vi "MT Generate PSK System Parameters(M).vi"(0 "samples per symbol (16)":i32=16, 1 "PSK type":u16(ring) items=["normal", "shifted", "offset"], 5 "M-PSK (4)":i32=4, 7 "differential PSK":enum16{"disable", "enable"}(ring), 11 "error in (no error)":errorcluster) -> (6 "PSK system parameters":T1 {"PSK type" items=["normal", "shifted", "offset"]; "symbol map" format="%.3f"}, 8 "bits per symbol":i32, 15 "error out":errorcluster)   [LabVIEW 2020, in "niDMT.lvlib"]
doc: "This polymorphic instance calculates parameters for use with either the MT Modulate PSK VI or the MT Demodulate PSK VI. This VI generates the symbol map for PSK-modulated systems. This VI accepts an M-ary value that specifies a predefined symbol map with the number of distinct symbol map values to use as symbols."
uses:
  <vilib>/addons/Modulation/niDMT.lvlib
  <vilib>/addons/Modulation/Digital/Support/Controls/PSK System Parameters.ctl
  <vilib>/addons/Modulation/niAMT.lvlib
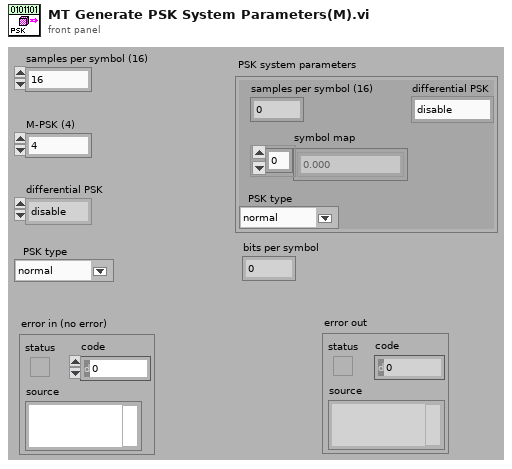
[diagram p1: front panel]
types:
  T1 = cluster{"samples per symbol (16)":i32, "symbol map":cdb[], "differential PSK":enum16{"disable", "enable"}, "PSK type":u16}
  T2 = typedef "niDMT.lvlib/PSK System Parameters.ctl" = cluster{"samples per symbol (16)":i32, "symbol map":cdb[], "differential PSK":enum16{"disable", "enable"}, "PSK type":u16}
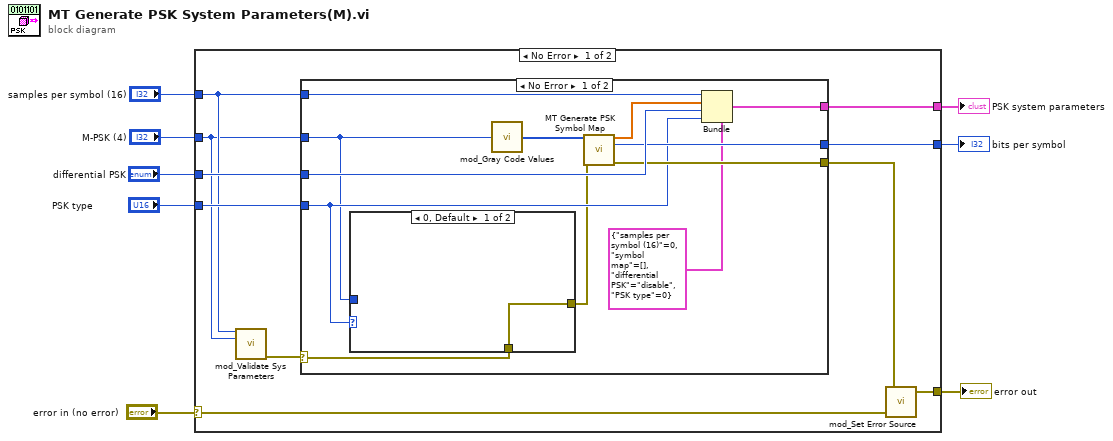
[diagram p0: block diagram]
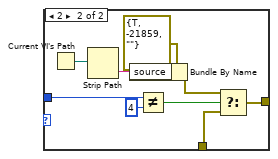
[diagram p2: hidden frame]
diagram:
  n1 = case shown="No Error" "error in (no error)" {
    selector: "error in (no error)" -> [w12 w42]
    tunnel: "samples per symbol (16)" -> [w10 _]
    tunnel: "differential PSK" -> [w18 _]
    tunnel: [w17 _] -> w6
    tunnel: "M-PSK (4)" -> [w9 _]
    tunnel: "PSK type" -> [w13 _]
    tunnel: [w16 _] -> w3
    tunnel: [w15 w42] -> w2
    frame No Error {
      n2 = call <vilib>:"mod_Validate Sys Parameters.vi"("samples per symbol"=w10, "M-ary"=w9) -> ("error out"=w11:errorcluster)  [unwired: 13 out]
      n3 = case shown="No Error" w11 {
        selector: w11 -> [w20 w41]
        tunnel: w18 -> [w30 _]
        tunnel: [w29 _] -> w17
        tunnel: [w26 _] -> w16
        tunnel: [w25 w41] -> w14
        tunnel: w13 -> [w24 _]
        tunnel: w9 -> [w23 _]
        tunnel: w10 -> [w21 _]
        frame No Error {
          n4 = case shown="0, Default" w24 {
            tunnel: w23 -> [_ w40]
            tunnel: w20 -> [w31 w37]
            tunnel: [w31 w36] -> w22
            frame 0, Default {
            }
            frame 2 {
              n5 = Current VI's Path() -> (path=w35:path)
              n6 = Strip Path(path=w35) -> (name=w33:string)  [unwired: 1 out]
              n7 = Bundle By Name(cluster=errorcluster {"status"=TRUE, "code"=-21859, "source"=""} ("error IO"), "source"=w33) -> (w32:errorcluster)
              n8 = Not Equal?(x=w40, y=4) -> (x != y?=w38:bool)
              n9 = Select(t=w32, s=w38, f=w37) -> (s? t:f=w36:errorcluster)
            }
          }
          n10 = call <vilib>:"mod_Gray Code Values.vi"("M"=w23) -> ("Gray coded values"=w27:i32[])
          n11 = call <vilib>:"MT Generate PSK Symbol Map.vi"("symbol values"=w27, "error in (no error)"=w22) -> ("symbol map"=w28:cdb[], "bits per symbol"=w26:i32, "error out"=w25:errorcluster)  [unwired: 11 out]
          n12 = Bundle(cluster=T2 {"samples per symbol (16)"=0, "symbol map"=[], "differential PSK"=enum."disable", "PSK type"=0} ("PSK system parameters"), "samples per symbol (16)"=w21, "symbol map"=w28, "differential PSK"=w30, "PSK type"=w24) -> (w29:T2)
        }
        frame Error {
        }
      }
      n13 = call <vilib>:"mod_Set Error Source.vi"("initial error in (no error)"=w12, "final error in (no error)"=w14) -> ("error out"=w15:errorcluster)  [unwired: 3 out]
    }
    frame Error {
    }
  }
  "PSK system parameters" <- w6
  "bits per symbol" <- w3
  "error out" <- w2
